vi "CRYPlot Curves Graph.vi"(10 "Rows In":i32[](array[numeric]), 11 "Graph Type":string) -> (2 "Curve Names Out":string[](array[string]), 3 "All Rows Out":i32[](array[numeric]))   [LabVIEW 2013]
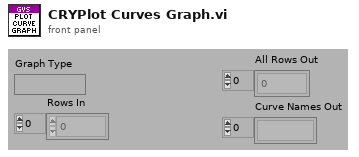
[diagram p1: front panel]
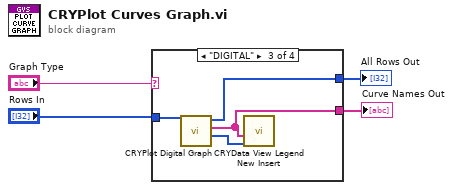
[diagram p0: block diagram]
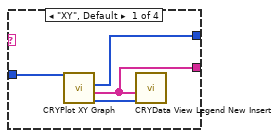
[diagram p2: hidden frame]
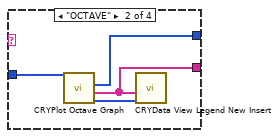
[diagram p3: hidden frame]
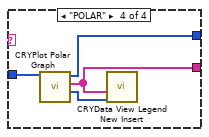
[diagram p4: hidden frame]
diagram:
  n1 = case shown="\"DIGITAL\"" "Graph Type" {
    tunnel: "Rows In" -> [w8 w12 w16 w20]
    tunnel: [w6 w10 w14 w19] -> w3
    tunnel: [w5 w9 w13 w18] -> w2
    frame "XY", Default {
      n2 = call "CRYPlot XY Graph.vi"("Selected Rows In"=w8) -> ("Color Info"=w7:u32[], "Curve Name"=w5:string[], "All Rows Out"=w6:i32[])  [unwired: 5 in, 3 out]
      n3 = call "CRYData View Legend New Insert.vi"("Color Array"=w7, "ItemName Array"=w5) -> ()  [unwired: 3 in, 7 out]
    }
    frame "OCTAVE" {
      n4 = call "CRYPlot Octave Graph.vi"("Selected Rows In"=w12) -> ("Color Info"=w11:u32[], "Curve Name"=w9:string[], "All Rows Out"=w10:i32[])  [unwired: 7 in, 1 out]
      n5 = call "CRYData View Legend New Insert.vi"("Color Array"=w11, "ItemName Array"=w9) -> ()  [unwired: 3 in, 7 out]
    }
    frame "DIGITAL" {
      n6 = call "CRYPlot Digital Graph.vi"("Selected Row In"=w16) -> ("Color Info"=w15:u32[], "Curve Name"=w13:string[], "Selected Row Out"=w14:i32[])  [unwired: 3 in, 5 out]
      n7 = call "CRYData View Legend New Insert.vi"("Color Array"=w15, "ItemName Array"=w13) -> ()  [unwired: 3 in, 7 out]
    }
    frame "POLAR" {
      n8 = call "CRYPlot Polar Graph.vi"("Selected Rows In"=w20) -> ("Freq Color"=w17:u32[], "Freq Name"=w18:string[], "Selected Row Out"=w19:i32[])  [unwired: 4 in, 4 out]
      n9 = call "CRYData View Legend New Insert.vi"("Color Array"=w17, "ItemName Array"=w18) -> ()  [unwired: 3 in, 7 out]
    }
  }
  "All Rows Out" <- w3
  "Curve Names Out" <- w2
